vi "celceus_to_farhrenheit.vi"() -> ()   [LabVIEW 2019]
panel:
  out "fahrenheit":dbl
  in  "celsius":dbl
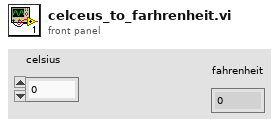
[diagram p1: front panel]
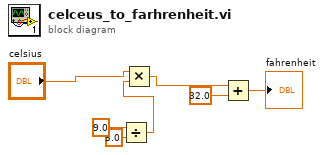
[diagram p0: block diagram]
diagram:
  n1 = Divide(x=9.0, y=5.0) -> (x/y=w7:dbl)
  n2 = Multiply(x="celsius", y=w7) -> (x*y=w3:dbl)
  n3 = Add(x=w3, y=32.0) -> (x+y=→"fahrenheit":dbl)
